vi "hardware_optpump_stirap.vi"(8 "error in":errorcluster, 10 "Pump?":bool) -> (0 "error out":errorcluster)   [LabVIEW 2012]
uses:
  <vilib>/DAQmx/write.llb/DAQmx Write (Digital Wfm 1Chan NSamp).vi
  <vilib>/Waveform/DWDTOps.llb/Digital Pattern Generator (Single Value).vi
  <vilib>/DAQmx/create/channels.llb/DAQmx Create Channel (DO-Digital Output).vi
  <vilib>/Waveform/DWDTOps.llb/DWDT Append Digital Samples.vi
  <vilib>/Waveform/DWDTOps.llb/DWDT Digital Size.vi
  <vilib>/DAQmx/configure/timing.llb/DAQmx Timing (Sample Clock).vi
  <vilib>/Waveform/DWDTOps.llb/DWDT Uncompress Digital.vi
  <vilib>/DAQmx/miscellaneous.llb/DAQmx Fill In Error Info.vi
  <resource>/objmgr/daqmx.rc
panel:
  out "error out 2":errorcluster
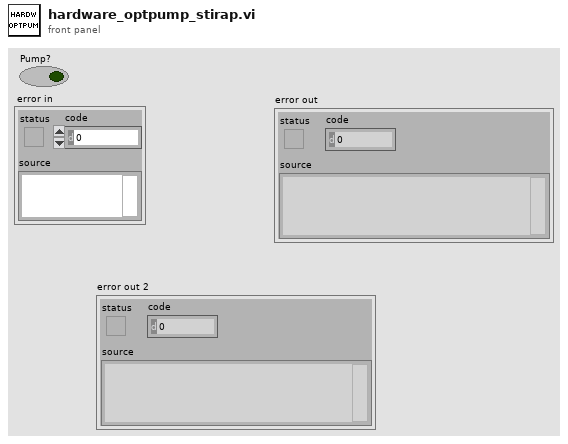
[diagram p1: front panel]
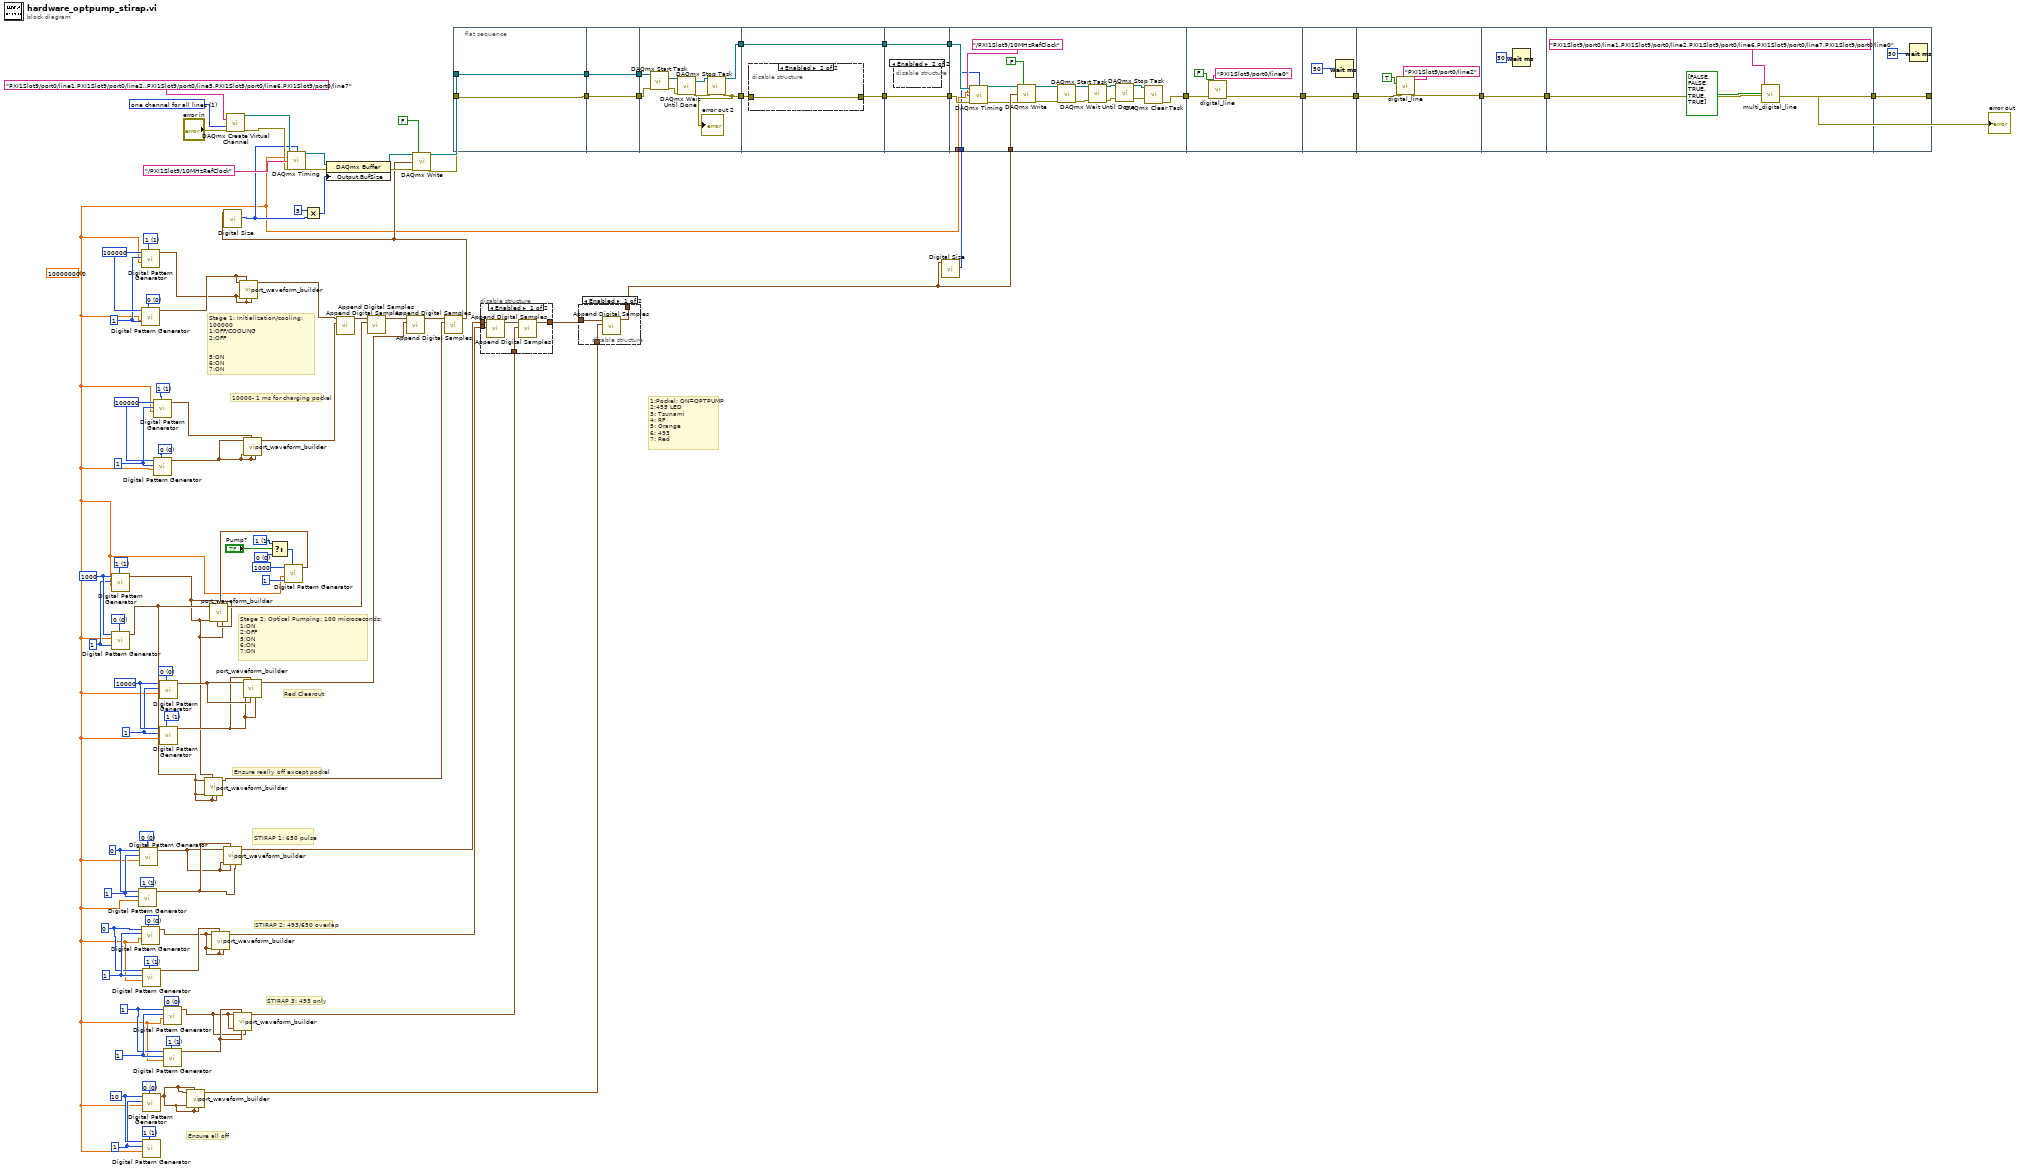
[diagram p0: block diagram]
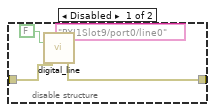
[diagram p4: hidden frame]
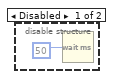
[diagram p5: hidden frame]
diagram:
  w15 = u32 1 ("number of samples")
  w18 = u8 1 items=["0", "1", "Z", "L", "H", "X", "T", "V"] ("value")
  w19 = u8 0 items=["0", "1", "Z", "L", "H", "X", "T", "V"] ("value")
  w20 = u32 1 ("number of signals")
  w21 = u32 0 ("number of samples")
  w22 = u8 1 items=["0", "1", "Z", "L", "H", "X", "T", "V"] ("value")
  w23 = u8 0 items=["0", "1", "Z", "L", "H", "X", "T", "V"] ("value")
  w24 = u32 1 ("number of signals")
  w48 = u8 0 items=["0", "1", "Z", "L", "H", "X", "T", "V"] ("value")
  w46 = u32 1 ("number of signals")
  w47 = u32 10000 ("number of samples")
  w49 = u8 1 items=["0", "1", "Z", "L", "H", "X", "T", "V"] ("value")
  w61 = u8 0 items=["0", "1", "Z", "L", "H", "X", "T", "V"] ("value")
  w59 = u32 1 ("number of signals")
  w60 = u32 100000 ("number of samples")
  w62 = u8 1 items=["0", "1", "Z", "L", "H", "X", "T", "V"] ("value")
  w68 = u8 1 items=["0", "1", "Z", "L", "H", "X", "T", "V"] ("value")
  w67 = u8 0 items=["0", "1", "Z", "L", "H", "X", "T", "V"] ("value")
  w79 = u8 0 items=["0", "1", "Z", "L", "H", "X", "T", "V"] ("value")
  w77 = u32 1 ("number of signals")
  w78 = u32 10 ("number of samples")
  w80 = u8 1 items=["0", "1", "Z", "L", "H", "X", "T", "V"] ("value")
  w83 = u8 0 items=["0", "1", "Z", "L", "H", "X", "T", "V"] ("value")
  w81 = u32 1 ("number of signals")
  w82 = u32 0 ("number of samples")
  w84 = u8 1 items=["0", "1", "Z", "L", "H", "X", "T", "V"] ("value")
  w89 = u8 0 items=["0", "1", "Z", "L", "H", "X", "T", "V"] ("value")
  w85 = u32 1 ("number of signals")
  w86 = u32 1000 ("number of samples")
  w90 = u8 1 items=["0", "1", "Z", "L", "H", "X", "T", "V"] ("value")
  w91 = u8 0 items=["0", "1", "Z", "L", "H", "X", "T", "V"] ("value")
  w87 = u32 1 ("number of signals")
  w88 = u32 100000 ("number of samples")
  w92 = u8 1 items=["0", "1", "Z", "L", "H", "X", "T", "V"] ("value")
  w97 = 1 items=["one channel for each line", "one channel for all lines"] ("line grouping")
  w14 = 10000000.0 ("rate")
  # "Red Clearout"
  # "10000- 1 ms for charging pockel"
  # "STIRAP 3: 493 only"
  # "STIRAP 2: 493/650 overlap"
  # "Ensure really off except pockel"
  # "Ensure all off"
  # "STIRAP 1: 650 pulse"
  # "Stage 2: Optical Pumping: 100 microseconds: \n1:ON\n2:OFF\n5:ON\n6:ON\n7:ON"
  # "Stage 1: Initialization/cooling: 100000\n1:OFF/COOLING\n2:OFF\n\n\n5:ON\n6:ON\n7:ON"
  # "1:Pockel: ON=OPTPUMP\n2:455 LED\n3: Tsunami\n4: RF\n5: Orange\n6: 493\n7: Red"
  n1 = call-poly <vilib>:"Digital Pattern Generator.vi"("value"=w90, "sample rate"=w14, "number of signals"=w85, "number of samples"=w86) -> ("digital waveform"=w25:digitalwaveform)  [unwired: 6 in, 1 out]
  n2 = call-poly <vilib>:"Digital Pattern Generator.vi"("value"=w89, "sample rate"=w14, "number of signals"=w85, "number of samples"=w86) -> ("digital waveform"=w53:digitalwaveform)  [unwired: 6 in, 1 out]
  n3 = call-poly <vilib>:"Digital Pattern Generator.vi"("value"=w84, "sample rate"=w14, "number of signals"=w81, "number of samples"=w82) -> ("digital waveform"=w13:digitalwaveform)  [unwired: 6 in, 1 out]
  n4 = call-poly <vilib>:"Digital Pattern Generator.vi"("value"=w83, "sample rate"=w14, "number of signals"=w81, "number of samples"=w82) -> ("digital waveform"=w12:digitalwaveform)  [unwired: 6 in, 1 out]
  n5 = call-poly <vilib>:"Digital Pattern Generator.vi"("value"=w92, "sample rate"=w14, "number of signals"=w87, "number of samples"=w88) -> ("digital waveform"=w70:digitalwaveform)  [unwired: 6 in, 1 out]
  n6 = call-poly <vilib>:"Digital Pattern Generator.vi"("value"=w91, "sample rate"=w14, "number of signals"=w87, "number of samples"=w88) -> ("digital waveform"=w71:digitalwaveform)  [unwired: 6 in, 1 out]
  n7 = call-poly <vilib>:"Digital Pattern Generator.vi"("value"=w23, "sample rate"=w14, "number of signals"=w24, "number of samples"=w21) -> ("digital waveform"=w2:digitalwaveform)  [unwired: 6 in, 1 out]
  n8 = call-poly <vilib>:"Digital Pattern Generator.vi"("value"=w22, "sample rate"=w14, "number of signals"=w24, "number of samples"=w21) -> ("digital waveform"=w3:digitalwaveform)  [unwired: 6 in, 1 out]
  n9 = call-poly <vilib>:"Digital Pattern Generator.vi"("value"=w79, "sample rate"=w14, "number of signals"=w77, "number of samples"=w78) -> ("digital waveform"=w50:digitalwaveform)  [unwired: 6 in, 1 out]
  n10 = call-poly <vilib>:"Digital Pattern Generator.vi"("value"=w80, "sample rate"=w14, "number of signals"=w77, "number of samples"=w78) -> ()  [unwired: 6 in, 2 out]
  n11 = call-poly <vilib>:"Digital Pattern Generator.vi"("value"=w62, "sample rate"=w14, "number of signals"=w59, "number of samples"=w60) -> ("digital waveform"=w58:digitalwaveform)  [unwired: 6 in, 1 out]
  n12 = call-poly <vilib>:"Digital Pattern Generator.vi"("value"=w61, "sample rate"=w14, "number of signals"=w59, "number of samples"=w60) -> ("digital waveform"=w57:digitalwaveform)  [unwired: 6 in, 1 out]
  n13 = call-poly <vilib>:"Digital Pattern Generator.vi"("value"=w48, "sample rate"=w14, "number of signals"=w46, "number of samples"=w47) -> ("digital waveform"=w43:digitalwaveform)  [unwired: 6 in, 1 out]
  n14 = call-poly <vilib>:"Digital Pattern Generator.vi"("value"=w49, "sample rate"=w14, "number of signals"=w46, "number of samples"=w47) -> ("digital waveform"=w42:digitalwaveform)  [unwired: 6 in, 1 out]
  n15 = call-poly <vilib>:"Digital Pattern Generator.vi"("value"=w19, "sample rate"=w14, "number of signals"=w20, "number of samples"=w15) -> ("digital waveform"=w16:digitalwaveform)  [unwired: 6 in, 1 out]
  n16 = call-poly <vilib>:"Digital Pattern Generator.vi"("value"=w18, "sample rate"=w14, "number of signals"=w20, "number of samples"=w15) -> ("digital waveform"=w17:digitalwaveform)  [unwired: 6 in, 1 out]
  n17 = call "port_waveform_builder.vi"("Line 7"=w50, "Line 6"=w50, "Line 1"=w50, "Line 5"=w50, "Line 2"=w50) -> ("digital waveform out"=w75:digitalwaveform)  [unwired: 6 in]
  n18 = call "port_waveform_builder.vi"("Line 7"=w53, "Line 6"=w53, "Line 1"=w25, "Line 5"=w53, "Line 2"=w53) -> ("digital waveform out"=w9:digitalwaveform)  [unwired: 6 in]
  n19 = call "port_waveform_builder.vi"("Line 7"=w2, "Line 6"=w2, "Line 1"=w3, "Line 5"=w2, "Line 2"=w2) -> ("digital waveform out"=w10:digitalwaveform)  [unwired: 6 in]
  n20 = call "port_waveform_builder.vi"("Line 7"=w13, "Line 6"=w12, "Line 1"=w13, "Line 5"=w12, "Line 2"=w12) -> ("digital waveform out"=w11:digitalwaveform)  [unwired: 6 in]
  n21 = call-poly <vilib>:"DAQmx Create Virtual Channel.vi"("lines"=tag "PXI1Slot9/port0/line1,PXI1Slot9/port0/line2,,PXI1Slot9/port0/line5,PXI1Slot9/port0/line6,PXI1Slot9/port0/line7", "line grouping"=w97, "error in"="error in") -> ("task out"=w98:refnum<k21>, "error out"=w95:errorcluster)  [unwired: 11 in]
  n22 = call "port_waveform_builder.vi"("Line 7"=w16, "Line 6"=w17, "Line 1"=w17, "Line 5"=w16, "Line 2"=w16) -> ("digital waveform out"=w7:digitalwaveform)  [unwired: 6 in]
  n23 = call "port_waveform_builder.vi"("Line 7"=w70, "Line 6"=w70, "Line 1"=w71, "Line 5"=w70, "Line 2"=w71) -> ("digital waveform out"=w56:digitalwaveform)  [unwired: 6 in]
  n24 = call "port_waveform_builder.vi"("Line 7"=w42, "Line 6"=w43, "Line 1"=w42, "Line 5"=w42, "Line 2"=w43) -> ("digital waveform out"=w44:digitalwaveform)  [unwired: 6 in]
  n25 = call "port_waveform_builder.vi"("Line 7"=w57, "Line 6"=w57, "Line 1"=w58, "Line 5"=w57, "Line 2"=w57) -> ("digital waveform out"=w55:digitalwaveform)  [unwired: 6 in]
  n26 = Select(t=w68, s="Pump?", f=w67) -> (s? t:f=w64:u8)
  n27 = call-poly <vilib>:"Digital Pattern Generator.vi"("value"=w64, "sample rate"=w14, "number of signals"=u32 1, "number of samples"=u32 1000) -> ("digital waveform"=w26:digitalwaveform)  [unwired: 6 in, 1 out]
  n28 = call "port_waveform_builder.vi"("Line 7"=w25, "Line 6"=w26, "Line 1"=w25, "Line 5"=w25, "Line 2"=w53) -> ("digital waveform out"=w76:digitalwaveform)  [unwired: 6 in]
  n29 = call-poly <vilib>:"Append Digital Samples.vi"("digital waveform B"=w55, "digital waveform A"=w56) -> ("digital waveform out"=w54:digitalwaveform)  [unwired: 8 in, 1 out]
  n30 = call-poly <vilib>:"Append Digital Samples.vi"("digital waveform B"=w76, "digital waveform A"=w54) -> ("digital waveform out"=w45:digitalwaveform)  [unwired: 8 in, 1 out]
  n31 = call-poly <vilib>:"Append Digital Samples.vi"("digital waveform B"=w44, "digital waveform A"=w45) -> ("digital waveform out"=w1:digitalwaveform)  [unwired: 8 in, 1 out]
  n32 = call-poly <vilib>:"Append Digital Samples.vi"("digital waveform B"=w9, "digital waveform A"=w1) -> ("digital waveform out"=w34:digitalwaveform)  [unwired: 8 in, 1 out]
  n33 = call-poly <vilib>:"Digital Size.vi"("digital waveform in"=w34) -> ("number of samples"=w29:i32)  [unwired: 7 in, 3 out]
  n34 = call-poly <vilib>:"DAQmx Timing.vi"("task/channels in"=w98, "samples per channel"=w29, "rate"=w14, "source"=tag "/PXI1Slot9/10MHzRefClock", "error in"=w95) -> ("task out"=w103:refnum<k21>, "error out"=w102:errorcluster)  [unwired: 9 in]
  n35 = Multiply(x=5, y=w29) -> (x*y=w36:i32)
  n36 = property class="DAQmx Buffer"(reference=w103, error in=w102, "Output.BufSize"=w36) -> (reference out=w100:refnum<k21>, error out=w94:errorcluster)
  n37 = call-poly <vilib>:"DAQmx Write.vi"("task/channels in"=w100, "auto start"=FALSE, "data"=w34, "error in"=w94) -> ("task out"=w99:refnum<k21>, "error out"=w93:errorcluster)  [unwired: 9 in, 1 out]
  n38 = flat-sequence {
    tunnel: w93 -> [w105]
    tunnel: w99 -> [w106]
    tunnel: [w106] -> w40
    tunnel: [w105] -> w37
    tunnel: w40 -> [w108]
    tunnel: [w108] -> w39
    tunnel: [w107] -> w38
    tunnel: w37 -> [w107]
    tunnel: w39 -> [w116]
    tunnel: w38 -> [w115]
    tunnel: [w113] -> w31
    tunnel: [w109] -> w30
    tunnel: [w119] -> w52
    tunnel: [w117] -> w32
    tunnel: w31 -> [w117]
    tunnel: w30 -> [w118]
    tunnel: w52 -> [w126]
    tunnel: [w126] -> w35
    tunnel: [w125] -> w33
    tunnel: w32 -> [w125]
    tunnel: w35 -> [w134]
    tunnel: [w135] -> w5
    tunnel: w33 -> [w131]
    tunnel: w28 -> [w145]
    tunnel: w14 -> [w130]
    tunnel: w27 -> [w128]
    tunnel: w5 -> [w146]
    tunnel: [w147] -> w4
    tunnel: w4 -> [w151]
    tunnel: [w151] -> w6
    tunnel: [w152] -> w51
    tunnel: w6 -> [w153]
    tunnel: w51 -> [w157]
    tunnel: [w157] -> w69
    tunnel: w69 -> [w161]
    tunnel: [w160] -> w41
    tunnel: [w163] -> w73
    tunnel: w41 -> [w163]
    frame #0 {
    }
    frame #1 {
    }
    frame #2 {
      n39 = call <vilib>:"DAQmx Start Task.vi"("task/channels in"=w116, "error in"=w115) -> ("task out"=w114:refnum<k21>, "error out"=w110:errorcluster)  [unwired: 12 in]
      n40 = call <vilib>:"DAQmx Wait Until Done.vi"("task/channels in"=w114, "error in"=w110) -> ("task out"=w111:refnum<k21>, "error out"=w112:errorcluster)  [unwired: 12 in]
      n41 = call <vilib>:"DAQmx Stop Task.vi"("task/channels in"=w111, "error in"=w112) -> ("task out"=w113:refnum<k21>, "error out"=w109:errorcluster)  [unwired: 12 in]
      "error out 2" <- w109
    }
    frame #3 {
      n42 = disable-structure shown="Enabled" {
        disable-tunnel: [w123 w124] -> w119
        disable-tunnel: w118 -> [w122 w124]
        frame Disabled {
          n43 = call "digital_line.vi"("error in"=w122, "Boolean"=FALSE, "lines"=tag "PXI1Slot9/port0/line0") -> ("error out"=w123:errorcluster)  [unwired: 4 in]
        }
        frame Enabled {
        }
      }
    }
    frame #4 {
      n44 = disable-structure shown="Enabled" {
        frame Disabled {
          n45 = Wait (ms)(milliseconds to wait=u32 50) -> ()  [unwired: 1 out]
        }
        frame Enabled {
        }
      }
    }
    frame #5 {
      n46 = call-poly <vilib>:"DAQmx Timing.vi"("task/channels in"=w131, "samples per channel"=w128, "rate"=w130, "source"=tag "/PXI1Slot9/10MHzRefClock", "error in"=w134) -> ("task out"=w132:refnum<k21>, "error out"=w133:errorcluster)  [unwired: 9 in]
      n47 = call-poly <vilib>:"DAQmx Write.vi"("task/channels in"=w132, "auto start"=FALSE, "data"=w145, "error in"=w133) -> ("task out"=w143:refnum<k21>, "error out"=w136:errorcluster)  [unwired: 9 in, 1 out]
      n48 = call <vilib>:"DAQmx Start Task.vi"("task/channels in"=w143, "error in"=w136) -> ("task out"=w142:refnum<k21>, "error out"=w137:errorcluster)  [unwired: 12 in]
      n49 = call <vilib>:"DAQmx Wait Until Done.vi"("task/channels in"=w142, "error in"=w137) -> ("task out"=w141:refnum<k21>, "error out"=w138:errorcluster)  [unwired: 12 in]
      n50 = call <vilib>:"DAQmx Stop Task.vi"("task/channels in"=w141, "error in"=w138) -> ("task out"=w140:refnum<k21>, "error out"=w139:errorcluster)  [unwired: 12 in]
      n51 = call <vilib>:"DAQmx Clear Task.vi"("task in"=w140, "error in"=w139) -> ("error out"=w135:errorcluster)  [unwired: 13 in]
    }
    frame #6 {
      n52 = call "digital_line.vi"("error in"=w146, "Boolean"=FALSE, "lines"=tag "PXI1Slot9/port0/line0") -> ("error out"=w147:errorcluster)  [unwired: 4 in]
    }
    frame #7 {
      n53 = Wait (ms)(milliseconds to wait=u32 50) -> ()  [unwired: 1 out]
    }
    frame #8 {
      n54 = call "digital_line.vi"("error in"=w153, "Boolean"=TRUE, "lines"=tag "PXI1Slot9/port0/line2") -> ("error out"=w152:errorcluster)  [unwired: 4 in]
    }
    frame #9 {
      n55 = Wait (ms)(milliseconds to wait=u32 50) -> ()  [unwired: 1 out]
    }
    frame #10 {
      n56 = call "multi_digital_line.vi"("error in"=w161, "data"=bool[] [FALSE, FALSE, TRUE, TRUE, TRUE], "lines"=tag "PXI1Slot9/port0/line1,PXI1Slot9/port0/line2,PXI1Slot9/port0/line6,PXI1Slot9/port0/line7,PXI1Slot9/port0/line0") -> ("error out"=w160:errorcluster)  [unwired: 8 in]
    }
    frame #11 {
      n57 = Wait (ms)(milliseconds to wait=u32 50) -> ()  [unwired: 1 out]
    }
  }
  n58 = disable-structure shown="Enabled" {
    disable-tunnel: w11 -> [w168 _]
    disable-tunnel: w10 -> [w167 _]
    disable-tunnel: [w165 w169] -> w8
    disable-tunnel: w7 -> [w164 w169]
    frame Enabled {
      n59 = call-poly <vilib>:"Append Digital Samples.vi"("digital waveform B"=w167, "digital waveform A"=w168) -> ("digital waveform out"=w166:digitalwaveform)  [unwired: 8 in, 1 out]
      n60 = call-poly <vilib>:"Append Digital Samples.vi"("digital waveform B"=w164, "digital waveform A"=w166) -> ("digital waveform out"=w165:digitalwaveform)  [unwired: 8 in, 1 out]
    }
    frame Disabled {
    }
  }
  n61 = disable-structure shown="Enabled" {
    disable-tunnel: w75 -> [w172 _]
    disable-tunnel: [w171 w173] -> w28
    disable-tunnel: w8 -> [w170 w173]
    frame Enabled {
      n62 = call-poly <vilib>:"Append Digital Samples.vi"("digital waveform B"=w172, "digital waveform A"=w170) -> ("digital waveform out"=w171:digitalwaveform)  [unwired: 8 in, 1 out]
    }
    frame Disabled {
    }
  }
  n63 = call-poly <vilib>:"Digital Size.vi"("digital waveform in"=w28) -> ("number of samples"=w27:i32)  [unwired: 7 in, 3 out]
  "error out" <- w73
